vi "Config Spark Max SLOT SmartMotion HW Get Set.vi"(4 "PIDF Slot (0)":i32, 6 "Get(f) Set(t)":bool, 7 "SparkMax Slot SM":T1={"Max Velocity"=0.0, "Max Acceleration"=1.0, "Allowed CL Error"=0.0, "Min Velocity Output"=0.0}, 8 "Error":errorcluster, 11 "Drive Refs":T2) -> (0 "Error Out":errorcluster, 3 "Drive Refs Out":T2, 5 "SparkMax Slot SM Out":T1={"Max Velocity"=0.0, "Max Acceleration"=1.0, "Allowed CL Error"=0.0, "Min Velocity Output"=0.0})   [LabVIEW 2023, in "Swerve-SteerSRX-DriveSpark-AbsAnalog_ACT.lvlib"]
uses:
  Swerve-SteerSRX-DriveSpark-AbsAnalog_ACT.lvlib
  <vilib>/Rock Robotics/WPI/MotorControl/WPI_MotorControlDeviceRef.ctl
  <vilib>/Rock Robotics/WPI/MotorControl/WPI_MotorControlType.ctl
  <vilib>/Rock Robotics/SystemInterfaces/DIO/FPGA_DIOPWMChannel.ctl
  <vilib>/Rock Robotics/WPI/PWM/WPI_PWMDeadband.ctl
  <vilib>/Rock Robotics/SystemInterfaces/DIO/FPGA_DIOChannel.ctl
  Shared Code/TypeDefs/Cluster_SparkMax Config_Smart Motion Parameters.ctl
  <vilib>/Utility/error.llb/Trim Whitespace One-Sided.vi
  <vilib>/Utility/Data Type/NI_Data Type.lvlib
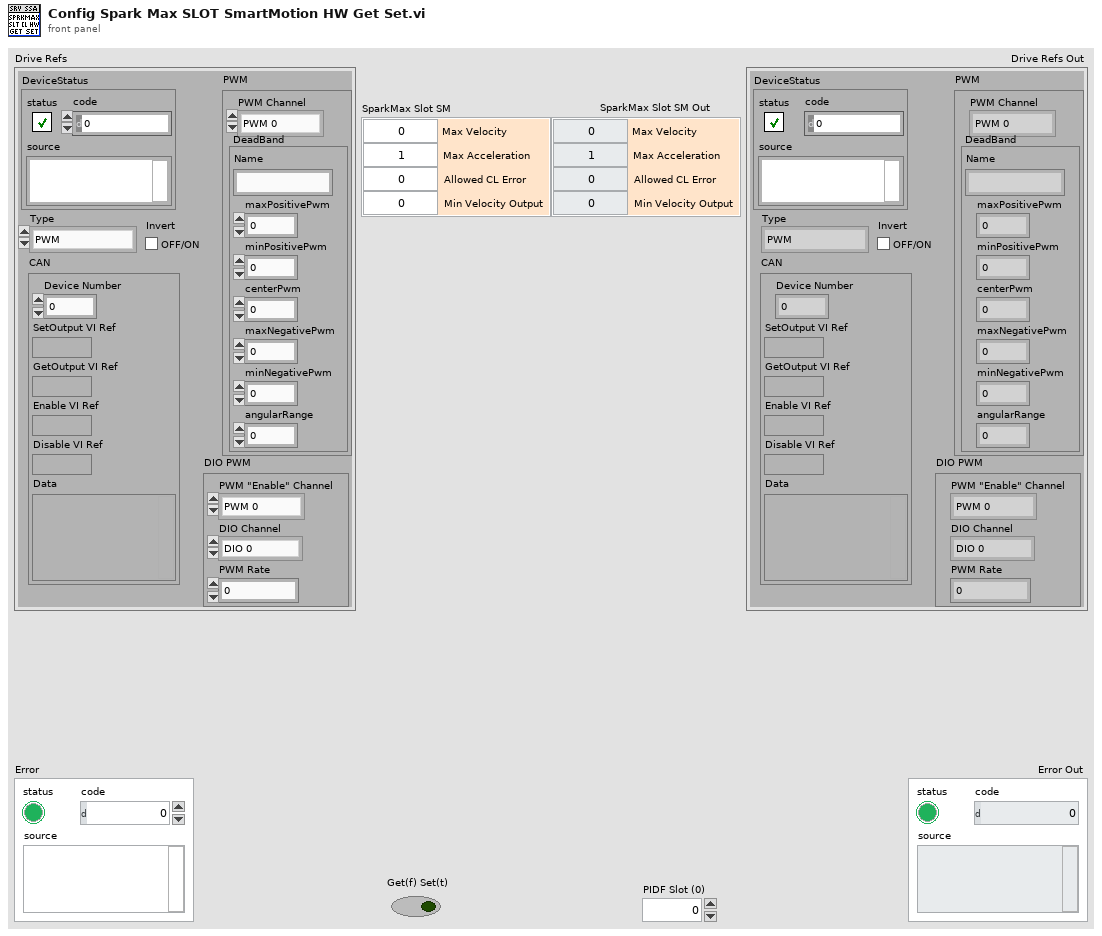
[diagram p1: front panel]
types:
  T1 = typedef "Cluster_SparkMax Config_Smart Motion Parameters.ctl" = cluster{"Max Velocity":dbl, "Max Acceleration":dbl, "Allowed CL Error":dbl, "Min Velocity Output":dbl}
  T2 = typedef "WPI_MotorControlDeviceRef.ctl" = cluster{"DeviceStatus":errorcluster, "Type":T3, "PWM":cluster{"PWM Channel":T4, "DeadBand":T5}, "CAN":cluster{"Device Number":u8, "SetOutput VI Ref":variant, "GetOutput VI Ref":variant, "Enable VI Ref":variant, "Disable VI Ref":variant, "Data":variant}, "Invert":bool, "DIO PWM":cluster{"PWM \"Enable\" Channel":T4, "DIOChannel":T6, "PWM Rate":dbl}}
  T3 = typedef "WPI_MotorControlType.ctl" = enum16{"PWM", "CAN", "DIO PWM"}
  T4 = typedef "FPGA_DIOPWMChannel.ctl" = enum8{"PWM 0", "PWM 1", "PWM 2", "PWM 3", "PWM 4", "PWM 5", "PWM 6", "PWM 7", "PWM 8", "PWM 9", "PWM MXP 0", "PWM MXP 1", "PWM MXP 2", "PWM MXP 3", "PWM MXP 4", "PWM MXP 5", "PWM MXP 6", "PWM MXP 7", "PWM MXP 8", "PWM MXP 9", "Invalid"}
  T5 = typedef "WPI_PWMDeadband.ctl" = cluster{"Name":string, "maxPositivePwm":i32, "minPositivePwm":i32, "centerPwm":i32, "maxNegativePwm":i32, "minNegativePwm":i32, "angularRange":u16}
  T6 = typedef "FPGA_DIOChannel.ctl" = enum8{"DIO 0", "DIO 1", "DIO 2", "DIO 3", "DIO 4", "DIO 5", "DIO 6", "DIO 7", "DIO 8", "DIO 9", "DIO MXP 0", "DIO MXP 1", "DIO MXP 2", "DIO MXP 3", "DIO MXP 4", "DIO MXP 5", "DIO MXP 6", "DIO MXP 7", "DIO MXP 8", "DIO MXP 9", "DIO MXP 10", "DIO MXP 11", "DIO MXP 12", "DIO MXP 13", "DIO MXP 14", "DIO MXP 15", "SPI Port CS1", "SPI Port CS2", "SPI Port CS3", "SPI Port MISO", "SPI Port MOSI", "Invalid"}
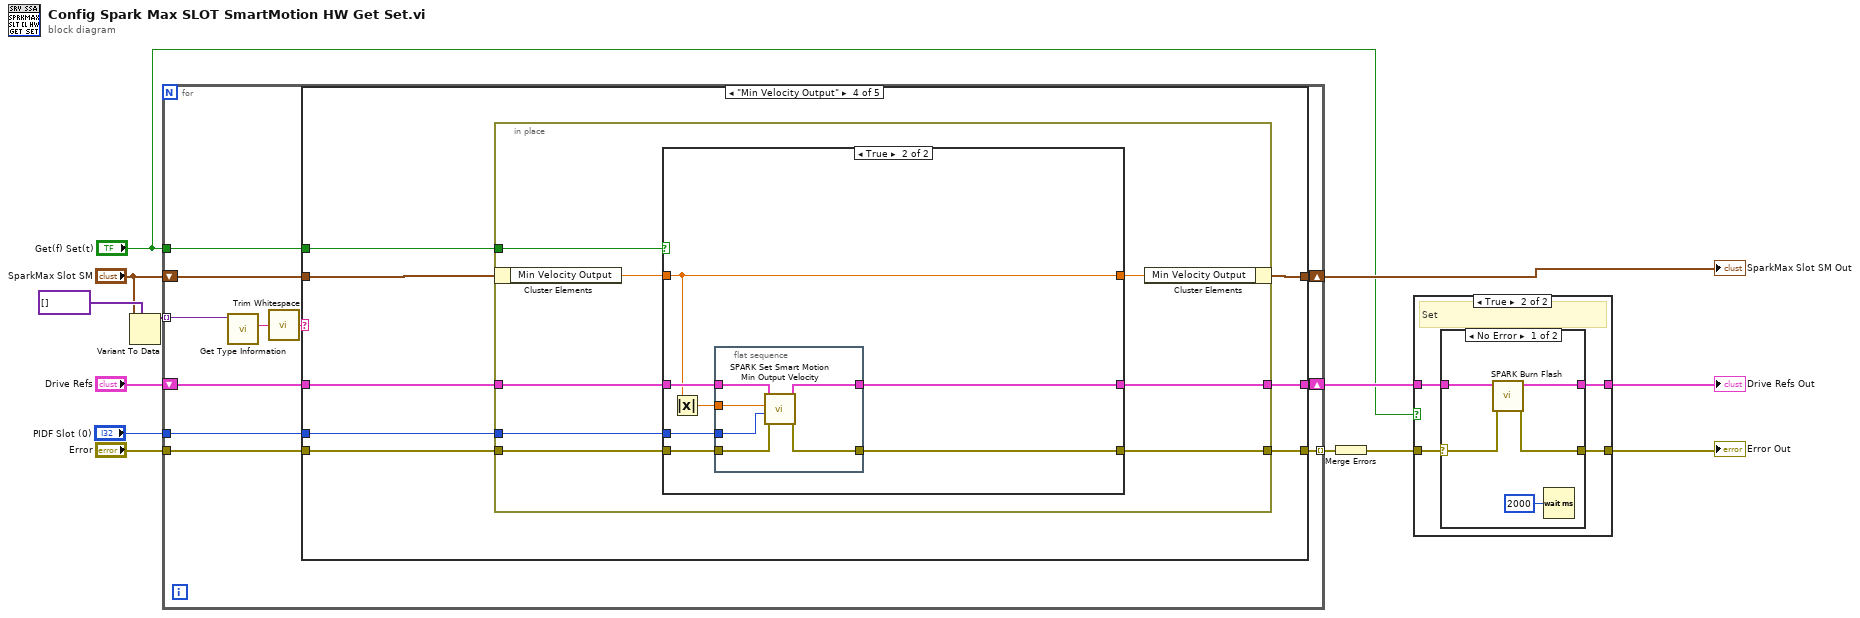
[diagram p0: block diagram]
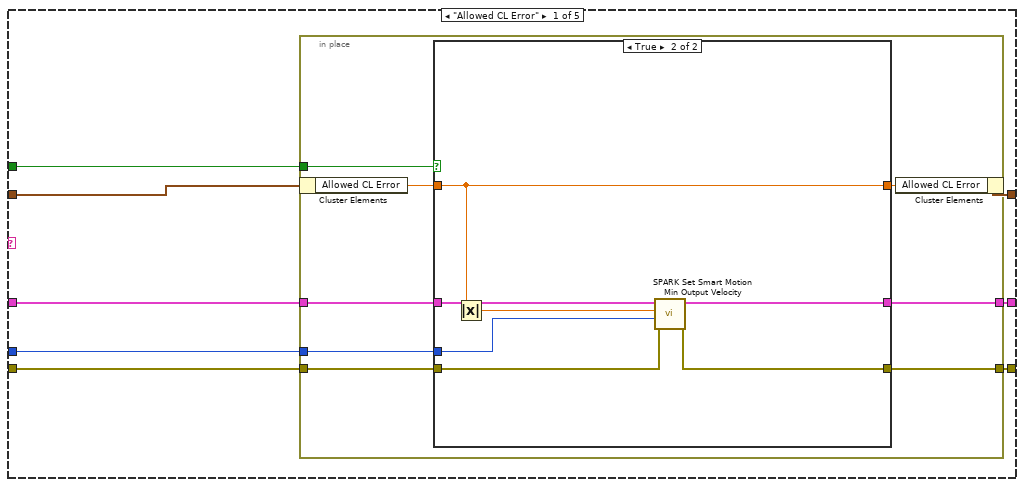
[diagram p4: hidden frame]
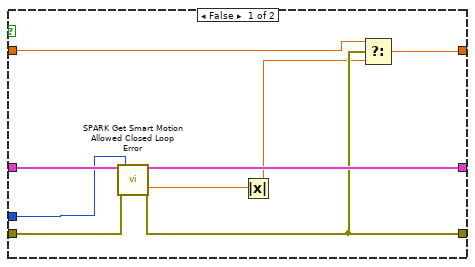
[diagram p5: hidden frame]
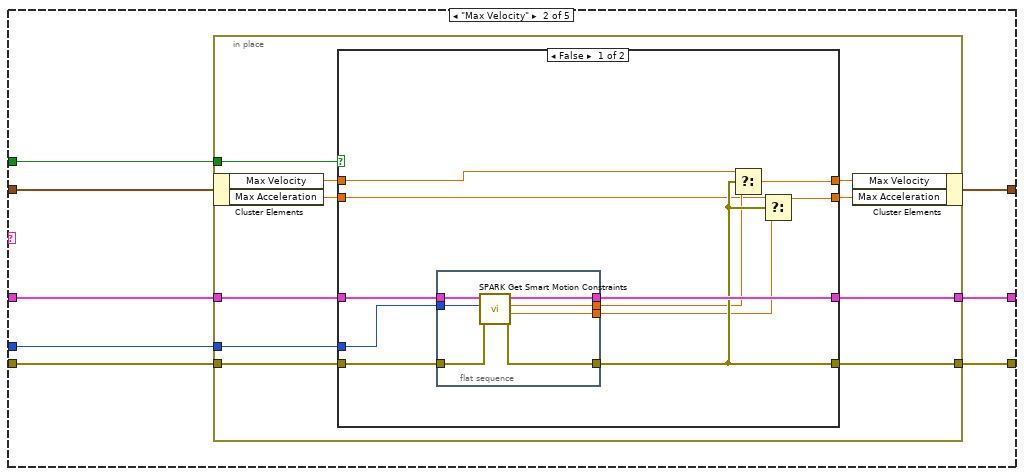
[diagram p6: hidden frame]
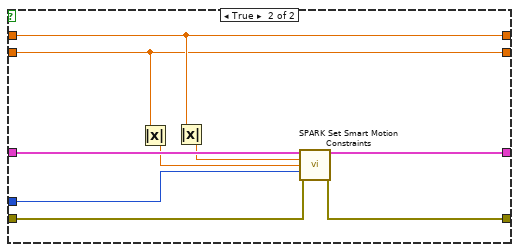
[diagram p7: hidden frame]
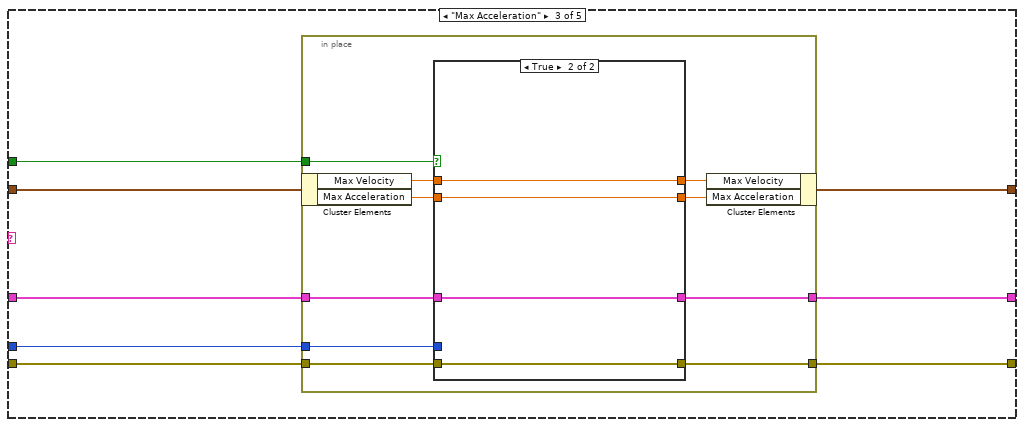
[diagram p8: hidden frame]
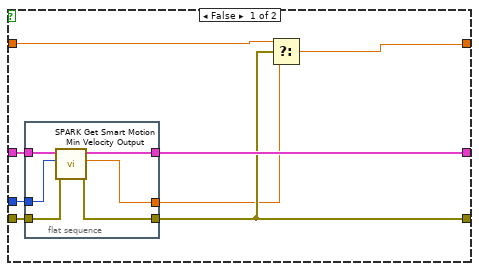
[diagram p10: hidden frame]
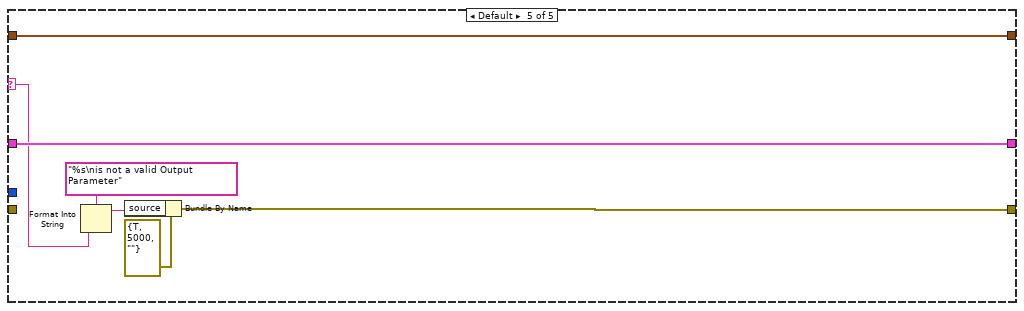
[diagram p11: hidden frame]
diagram:
  n1 = Variant To Data(type=variant[] [], Variant="SparkMax Slot SM") -> (data=w10:variant[])  [unwired: 1 in, 1 out]
  n2 = for {
    shift-right: [w15] -> w13
    shift-left: "SparkMax Slot SM" -> [w21]
    shift-right: [w16] -> w3
    shift-left: "Drive Refs" -> [w20]
    tunnel: "Get(f) Set(t)" -> [w19]
    tunnel: w10 -> [w23] mode=indexing
    tunnel: "Error" -> [w18]
    tunnel: [w17] -> w7 mode=indexing
    tunnel: "PIDF Slot (0)" -> [w14]
    n3 = call <vilib>:"Get Type Information.vi"("variant"=w23) -> ("name"=w24:string)  [unwired: 6 in, 4 out]
    n4 = call <vilib>:"Trim Whitespace.vi"("string"=w24) -> ("trimmed string"=w22:string)  [unwired: 1 in]
    n5 = case shown="\"Min Velocity Output\"" w22 {
      selector: w22 -> [_ _ _ _ w175]
      tunnel: w21 -> [w32 w64 w109 w135 w177]
      tunnel: w20 -> [w28 w60 w105 w131 w176]
      tunnel: w19 -> [w31 w63 w108 w134 _]
      tunnel: w18 -> [w30 w62 w107 w133 _]
      tunnel: [w29 w61 w106 w132 w173] -> w17
      tunnel: [w27 w59 w104 w130 w176] -> w16
      tunnel: [w26 w58 w103 w129 w177] -> w15
      tunnel: w14 -> [w25 w57 w102 w128 _]
      frame "Allowed CL Error" {
        n6 = in-place {
          in-place-border: w31 -> [w40]
          in-place-border: w30 -> [w38]
          in-place-border: [w37] -> w29
          in-place-border: w28 -> [w36]
          in-place-border: [w35] -> w27
          in-place-border: w25 -> [w33]
          n7 = in-place-cluster #1(w32) -> ("Allowed CL Error"=w39:dbl)
          n8 = case shown="True" w40 {
            tunnel: w39 -> [w43 w56]
            tunnel: w38 -> [w45 w53]
            tunnel: [w44 w52] -> w37
            tunnel: w36 -> [w47 w55]
            tunnel: [w48 w54] -> w35
            tunnel: [w49 w56] -> w34
            tunnel: w33 -> [w46 w51]
            frame False {
              n9 = call <vilib>:"SPARK Get Smart Motion Allowed Closed Loop Error.vi"("MotorControlDeviceRef"=w47, "error in"=w45, "PIDF Slot (0)"=w46) -> ("MotorControlDeviceRef"=w48:T2, "Allowed Closed Loop Error"=w42:dbl, "error out"=w44:errorcluster)  [unwired: 14 in]
              n10 = Absolute Value(x=w42) -> (abs(x)=w41:dbl)
              n11 = Select(t=w43, s=w44, f=w41) -> (s? t:f=w49:dbl)
            }
            frame True {
              n12 = Absolute Value(x=w56) -> (abs(x)=w50:dbl)
              n13 = call <vilib>:"SPARK Set Smart Motion Min Output Velocity.vi"("error in"=w53, "PIDF Slot (0)"=w51, "Minimum Velocity Output"=w50, "MotorControlDeviceRef"=w55) -> ("error out"=w52:errorcluster, "MotorControlDeviceRef"=w54:T2)  [unwired: 6 in]
            }
          }
          n14 = in-place-cluster #1("Allowed CL Error"=w34) -> (w26:T1)
        }
      }
      frame "Max Velocity" {
        n15 = in-place {
          in-place-border: w63 -> [w74]
          in-place-border: w62 -> [w72]
          in-place-border: [w71] -> w61
          in-place-border: w60 -> [w70]
          in-place-border: [w69] -> w59
          in-place-border: w57 -> [w67]
          n16 = in-place-cluster #2(w64) -> ("Max Velocity"=w73:dbl, "Max Acceleration"=w66:dbl)
          n17 = case shown="False" w74 {
            tunnel: w73 -> [w76 w101]
            tunnel: w72 -> [w83 w98]
            tunnel: [w81 w97] -> w71
            tunnel: w70 -> [w85 w100]
            tunnel: [w84 w99] -> w69
            tunnel: [w77 w101] -> w68
            tunnel: w67 -> [w82 w94]
            tunnel: w66 -> [w75 w93]
            tunnel: [w79 w93] -> w65
            frame False {
              n18 = flat-sequence {
                tunnel: w85 -> [w91]
                tunnel: [w92] -> w84
                tunnel: w83 -> [w86]
                tunnel: w82 -> [w90]
                tunnel: [w87] -> w81
                tunnel: [w88] -> w80
                tunnel: [w89] -> w78
                frame #0 {
                  n19 = call <vilib>:"SPARK Get Smart Motion Constraints.vi"("error in"=w86, "PIDF Slot (0)"=w90, "MotorControlDeviceRef"=w91) -> ("error out"=w87:errorcluster, "Max Acceleration"=w88:dbl, "Max Velocity"=w89:dbl, "MotorControlDeviceRef"=w92:T2)  [unwired: 5 in]
                }
              }
              n20 = Select(t=w76, s=w81, f=w78) -> (s? t:f=w77:dbl)
              n21 = Select(t=w75, s=w81, f=w80) -> (s? t:f=w79:dbl)
            }
            frame True {
              n22 = Absolute Value(x=w93) -> (abs(x)=w95:dbl)
              n23 = Absolute Value(x=w101) -> (abs(x)=w96:dbl)
              n24 = call <vilib>:"SPARK Set Smart Motion Constraints.vi"("MotorControlDeviceRef"=w100, "Max Velocity"=w96, "Max Acceleration"=w95, "PIDF Slot (0)"=w94, "error in"=w98) -> ("MotorControlDeviceRef"=w99:T2, "error out"=w97:errorcluster)  [unwired: 9 in]
            }
          }
          n25 = in-place-cluster #2("Max Velocity"=w68, "Max Acceleration"=w65) -> (w58:T1)
        }
      }
      frame "Max Acceleration" {
        n26 = in-place {
          in-place-border: w108 -> [w119]
          in-place-border: w107 -> [w117]
          in-place-border: [w116] -> w106
          in-place-border: w105 -> [w115]
          in-place-border: [w114] -> w104
          in-place-border: w102 -> [w112]
          n27 = in-place-cluster #3(w109) -> ("Max Velocity"=w118:dbl, "Max Acceleration"=w111:dbl)
          n28 = case shown="True" w119 {
            tunnel: w118 -> [w123 w127]
            tunnel: w117 -> [w121 w124]
            tunnel: [w121 w124] -> w116
            tunnel: w115 -> [w120 w125]
            tunnel: [w120 w125] -> w114
            tunnel: [w123 w127] -> w113
            tunnel: w112 -> [_ _]
            tunnel: w111 -> [w122 w126]
            tunnel: [w122 w126] -> w110
            frame False {
            }
            frame True {
            }
          }
          n29 = in-place-cluster #3("Max Velocity"=w113, "Max Acceleration"=w110) -> (w103:T1)
        }
      }
      frame "Min Velocity Output" {
        n30 = in-place {
          in-place-border: w134 -> [w143]
          in-place-border: w133 -> [w141]
          in-place-border: [w140] -> w132
          in-place-border: w131 -> [w139]
          in-place-border: [w138] -> w130
          in-place-border: w128 -> [w136]
          n31 = in-place-cluster #4(w135) -> ("Min Velocity Output"=w142:dbl)
          n32 = case shown="True" w143 {
            tunnel: w142 -> [w150 w158]
            tunnel: w141 -> [w147 w164]
            tunnel: [w146 w163] -> w140
            tunnel: w139 -> [w149 w161]
            tunnel: [w148 w160] -> w138
            tunnel: [w151 w158] -> w137
            tunnel: w136 -> [w145 w162]
            frame False {
              n33 = flat-sequence {
                tunnel: w149 -> [w155]
                tunnel: [w156] -> w148
                tunnel: w147 -> [w153]
                tunnel: [w152] -> w146
                tunnel: w145 -> [w157]
                tunnel: [w154] -> w144
                frame #0 {
                  n34 = call <vilib>:"SPARK Get Smart Motion Min Velocity Output.vi"("error in"=w153, "PIDF Slot (0)"=w157, "MotorControlDeviceRef"=w155) -> ("error out"=w152:errorcluster, "Minimum Velocity Output"=w154:dbl, "MotorControlDeviceRef"=w156:T2)  [unwired: 6 in]
                }
              }
              n35 = Select(t=w150, s=w146, f=w144) -> (s? t:f=w151:dbl)
            }
            frame True {
              n36 = Absolute Value(x=w158) -> (abs(x)=w159:dbl)
              n37 = flat-sequence {
                tunnel: w164 -> [w165]
                tunnel: [w166] -> w163
                tunnel: w162 -> [w167]
                tunnel: w161 -> [w168]
                tunnel: [w169] -> w160
                tunnel: w159 -> [w170]
                frame #0 {
                  n38 = call <vilib>:"SPARK Set Smart Motion Min Output Velocity.vi"("error in"=w165, "PIDF Slot (0)"=w167, "Minimum Velocity Output"=w170, "MotorControlDeviceRef"=w168) -> ("error out"=w166:errorcluster, "MotorControlDeviceRef"=w169:T2)  [unwired: 6 in]
                }
              }
            }
          }
          n39 = in-place-cluster #4("Min Velocity Output"=w137) -> (w129:T1)
        }
      }
      frame Default {
        n40 = Format Into String(format string="%s\nis not a valid Output Parameter", w175) -> (resulting string=w171:string)  [unwired: 2 in, 1 out]
        n41 = Bundle By Name(cluster=errorcluster {"status"=TRUE, "code"=5000, "source"=""} ("error out"), "source"=w171) -> (w173:errorcluster)
      }
    }
  }
  "SparkMax Slot SM Out" <- w13
  n42 = Merge Errors(w7) -> (w5:errorcluster)
  n43 = case shown="True" "Get(f) Set(t)" {
    tunnel: w5 -> [w178 w183]
    tunnel: [w178 w182] -> w4
    tunnel: w3 -> [w179 w181]
    tunnel: [w179 w180] -> w2
    frame False {
      # "Get"
    }
    frame True {
      # "Set"
      n44 = case shown="No Error" w183 {
        selector: w183 -> [w188 w189]
        tunnel: [w187 w189] -> w182
        tunnel: w181 -> [w184 w190]
        tunnel: [w185 w190] -> w180
        frame No Error {
          n45 = call <vilib>:"SPARK Burn Flash.vi"("error in"=w188, "MotorControlDeviceRef"=w184) -> ("error out"=w187:errorcluster, "MotorControlDeviceRef"=w185:T2)  [unwired: 8 in]
          n46 = Wait (ms)(milliseconds to wait=u32 2000) -> ()  [unwired: 1 out]
        }
        frame Error {
        }
      }
    }
  }
  "Error Out" <- w4
  "Drive Refs Out" <- w2
